vi "Laguerre Pre Decon Mat LV.vi"(0 "laguerreBasis_array in":dbl[](array[numeric]), 1 "laguerreOrder":u64=12, 2 "dataLength":u64=680, 3 "error in (no error)":errorcluster, 5 "vv_array in":dbl[](array[numeric]), 7 "D_mat_array in":dbl[](array[numeric]), 9 "LHS_multiplier_array in":dbl[](array[numeric]), 11 "RHS_multiplier_array in":dbl[](array[numeric]), 12 "alpha":dbl=0.916, 13 "iRF_array":dbl[](array[numeric])) -> (4 "laguerreBasis_array out":dbl[](array[numeric]), 6 "vv_array out":dbl[](array[numeric]), 8 "D_mat_array out":dbl[](array[numeric]), 10 "LHS_multiplier_array out":dbl[](array[numeric]), 14 "error out":errorcluster, 15 "RHS_multiplier_array out":dbl[](array[numeric]))   [LabVIEW 2024, in "LaguerreDeconLib.lvlib"]
doc: "extern \"C\" DECONLIBRARY_API void LaguerrePreDeconMatLV(const unsigned long long laguerreOrder, const unsigned long long dataLength, const double alpha, const double* iRF_array, const unsigned long long iRF_length,\n double* laguerreBasis_array, unsigned long long* rows1, unsigned long long* cols1,\n double* vv_array, unsigned long long* rows2, unsigned long long* cols2,\n double* D_mat_array, unsigned long long* rows3, unsigned long long* cols3,\n double* LHS_multiplier_array, unsigned long long* rows4, unsigned long long* cols4,\n double* RHS_multiplier_array, unsigned long long* rows5, unsigned long long* cols5);"
uses:
  LaguerreDeconLib.lvlib
  LaguerreDeconDLL.dll
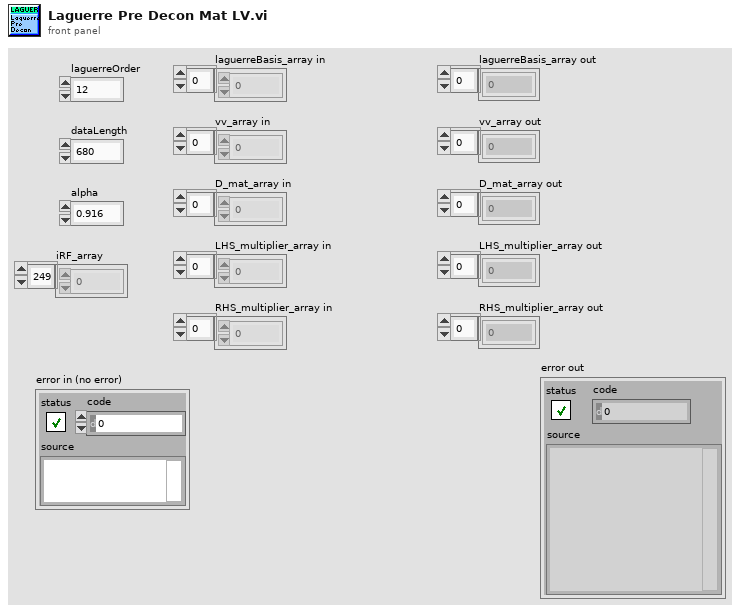
[diagram p1: front panel]
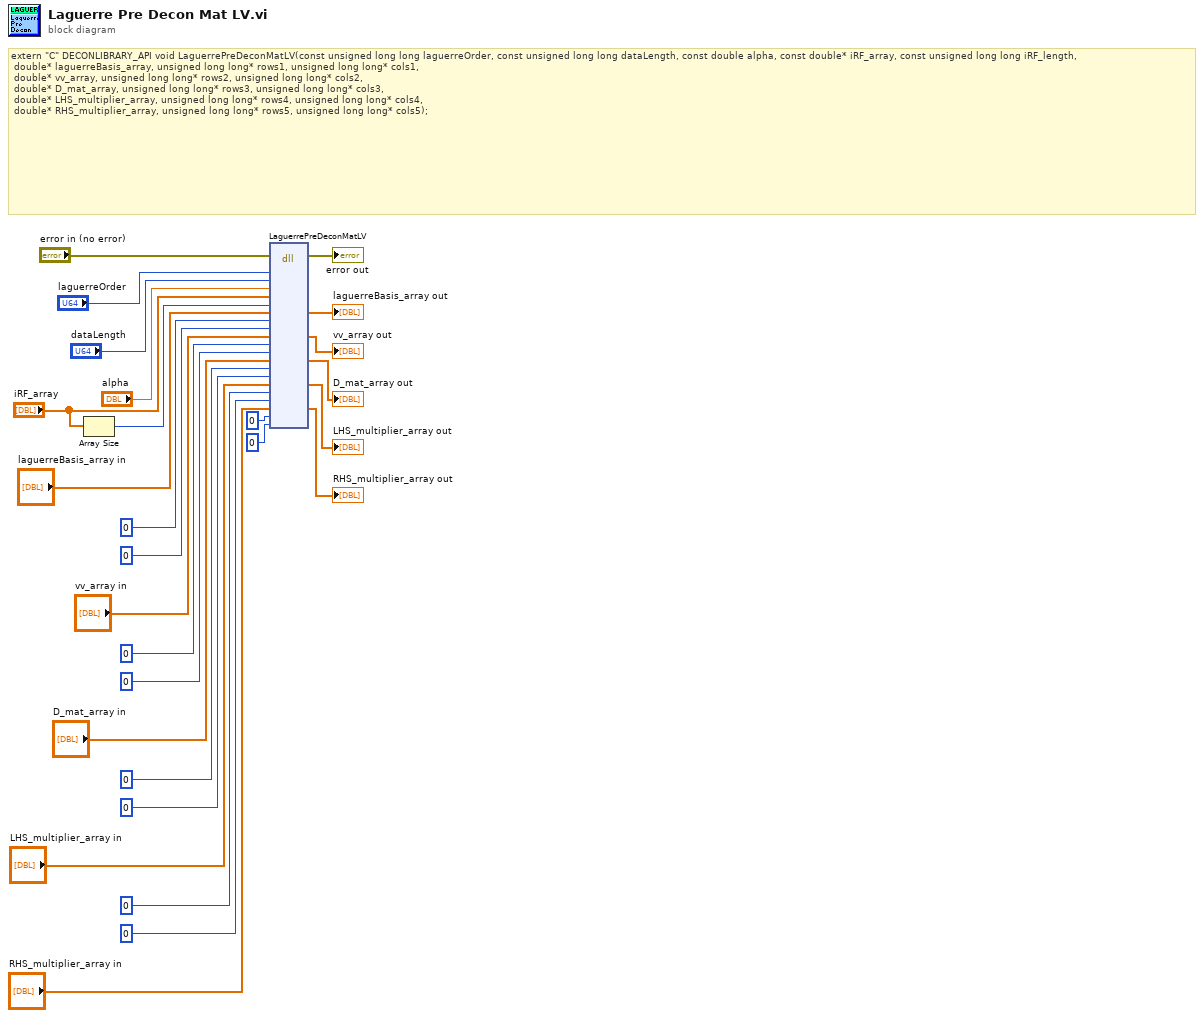
[diagram p0: block diagram]
diagram:
  # "extern \"C\" DECONLIBRARY_API void LaguerrePreDeconMatLV(const unsigned long long laguerreOrder, const unsigned long long dataLength, const double alpha, const double* iRF_array, const unsigned long long iRF_length,\n\tdouble* laguerreBasis_array, unsigned long long* rows1, unsigned long long* cols1,\n\tdouble* vv_array, unsigned long long* rows2, unsigned long long* cols2,\n\tdouble* D_mat_array, unsigned long long* rows3, unsigned long long* cols3,\n\tdouble* LHS_multiplier_array, unsigned long long* rows4, unsigned long long* cols4,\n\tdouble* RHS_multiplier_array, unsigned long long* rows5, unsigned long long* cols5);"
  n1 = Array Size(array="iRF_array") -> (size(s)=w17:i32)
  n2 = dll-call lib="C:/Users/MarcuAdmin/Documents/GitHub/FLSLV/V6 APD LV/LaguerreDeconLib/LaguerreDeconDLL.dll" fn="LaguerrePreDeconMatLV"(error in="error in (no error)", "laguerreOrder"="laguerreOrder", "dataLength"="dataLength", "alpha"="alpha", "iRF_array"="iRF_array", "iRF_length"=w17, "laguerreBasis_array"="laguerreBasis_array in", "rows1"=u64 0, "cols1"=u64 0, "vv_array"="vv_array in", "rows2"=u64 0, "cols2"=u64 0, "D_mat_array"="D_mat_array in", "rows3"=u64 0, "cols3"=u64 0, "LHS_multiplier_array"="LHS_multiplier_array in", "rows4"=u64 0, "cols4"=u64 0, "RHS_multiplier_array"="RHS_multiplier_array in", "rows5"=u64 0, "cols5"=u64 0) -> (error out=→"error out":errorcluster, "laguerreBasis_array"=→"laguerreBasis_array out":dbl[], "vv_array"=→"vv_array out":dbl[], "D_mat_array"=→"D_mat_array out":dbl[], "LHS_multiplier_array"=→"LHS_multiplier_array out":dbl[], "RHS_multiplier_array"=→"RHS_multiplier_array out":dbl[])  [unwired: 18 in, 1 out]
